vi "Handle Message.vi"(6 "Data":string, 8 "error in (no error)":errorcluster, 9 "Function ID":u8, 10 "Stack ID":u8, 11 "IP Connection in":refnum<class "IP Connection.lvclass">) -> (0 "error out":errorcluster, 3 "IP Connection out":refnum<class "IP Connection.lvclass">)   [LabVIEW 2011, in "Tinkerforge.lvlib" / "IP Connection.lvclass"]
doc: "This VI handles incoming messages."
uses:
  IP Connection.lvclass
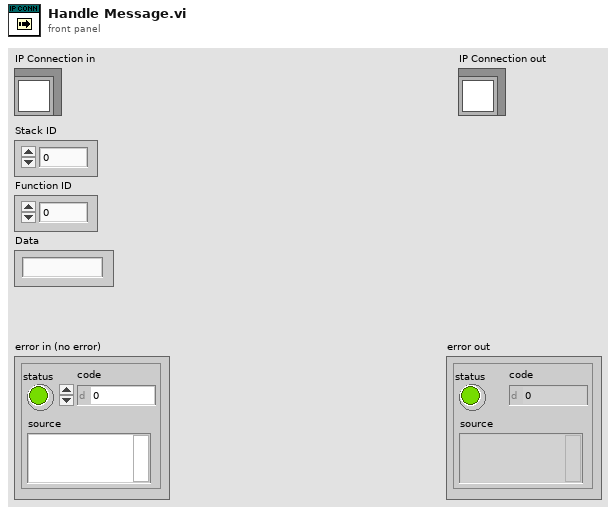
[diagram p1: front panel]
types:
  T1 = typedef "Tinkerforge.lvlib/IP Connection.lvclass/Functions.ctl" = enum8{"no Global Function", "get stack id", "enumerate", "CB enumerate"}
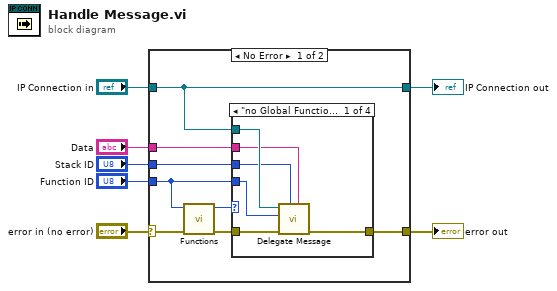
[diagram p0: block diagram]
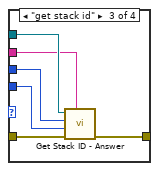
[diagram p3: hidden frame]
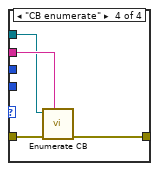
[diagram p4: hidden frame]
diagram:
  n1 = case shown="No Error" "error in (no error)" {
    selector: "error in (no error)" -> [w15 w34]
    tunnel: [w8 w34] -> w6
    tunnel: [w11 w33] -> w4
    tunnel: "IP Connection in" -> [w11 w33]
    tunnel: "Function ID" -> [w10 _]
    tunnel: "Stack ID" -> [w13 _]
    tunnel: "Data" -> [w12 _]
    frame No Error {
      n2 = call "Functions.vi"("Error In"=w15, "Function ID in"=w10) -> ("Error Out"=w14:errorcluster, "Function out"=w9:T1)  [unwired: 7 in, 1 out]
      n3 = case shown="\"no Global Function\"" w9 {
        tunnel: w14 -> [w21 w22 w28 w32]
        tunnel: w13 -> [w19 _ w25 _]
        tunnel: w12 -> [w18 _ w26 w31]
        tunnel: w10 -> [w17 _ w24 _]
        tunnel: w11 -> [w20 _ w27 w30]
        tunnel: [w16 w22 w23 w29] -> w8
        frame "no Global Function" {
          n4 = call "Delegate Message.vi"("Data"=w18, "Stack ID"=w19, "error in (no error)"=w21, "Function ID"=w17, "IP Connection in"=w20) -> ("error out"=w16:errorcluster)  [unwired: 5 in, 1 out]
        }
        frame Default {
        }
        frame "get stack id" {
          n5 = call "Get Stack ID - Answer.vi"("Data"=w26, "error in (no error)"=w28, "Function ID"=w24, "Stack ID"=w25, "IP Connection in"=w27) -> ("error out"=w23:errorcluster)  [unwired: 4 in, 2 out]
        }
        frame "CB enumerate" {
          n6 = call "Enumerate CB.vi"("Data"=w31, "error in (no error)"=w32, "IP Connection in"=w30) -> ("error out"=w29:errorcluster)  [unwired: 6 in, 2 out]
        }
      }
    }
    frame Error {
    }
  }
  "error out" <- w6
  "IP Connection out" <- w4
